vi "DLPIO20_Latch_Relay.vi"(6 "ON/OFF":bool, 7 "Relay":u16(ring) items=["RLY1"=1, "RLY2"=2], 8 "error in (no error)":errorcluster, 11 "VISA resource name":refnum<visa-resource-name>) -> (0 "error out":errorcluster, 3 "VISA resource name out":refnum<visa-resource-name>)   [LabVIEW 2016, in "DLPIO20_PackedLibrary.lvlib"]
uses:
  DLPIO20_PackedLibrary.lvlib
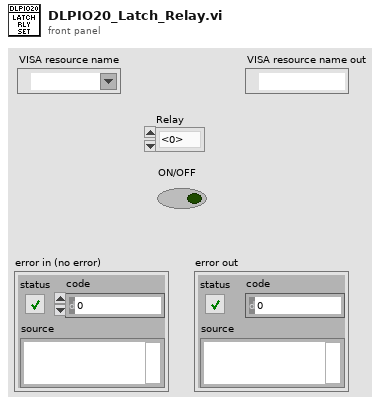
[diagram p1: front panel]
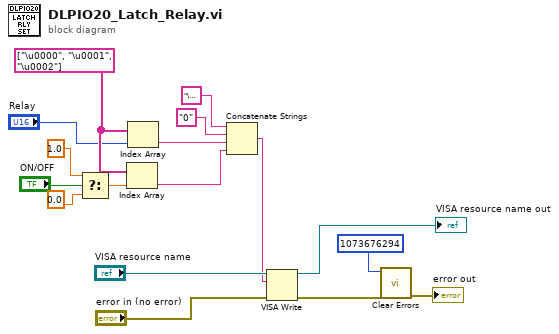
[diagram p0: block diagram]
diagram:
  w5 = string[] ["\u0000", "\u0001", "\u0002"]
  n1 = Select(t=1.0, s="ON/OFF", f=0.0) -> (s? t:f=w9:dbl)
  n2 = Index Array(array=w5, index=w9) -> (element=w2:string)
  n3 = Index Array(array=w5, index="Relay") -> (element=w3:string)
  n4 = Concatenate Strings("\u0004" ("string"), "0" ("string"), w3, w2) -> (w4:string)
  n5 = VISA Write(VISA resource name="VISA resource name", write buffer=w4, error in (no error)="error in (no error)") -> (VISA resource name out=→"VISA resource name out":refnum<visa-resource-name>, error out=w15:errorcluster)  [unwired: 1 out]
  n6 = call <vilib>:"Clear Errors.vi"("error in (no error)"=w15, "specific error code to clear (0: all)"=1073676294) -> ("error out"=→"error out":errorcluster)  [unwired: 4 in, 1 out]
